vi "WFM MNGR Initialize RF Waveforms.vi"(8 "error in (no error)":errorcluster, 10 "Sequence File":refnum<k7>, 11 "WFM MNGR in":refnum<class "QPA MSMT Waveform Manager.lvclass">) -> (0 "error out":errorcluster, 3 "WFM MNGR out":refnum<class "QPA MSMT Waveform Manager.lvclass">)   [LabVIEW 2016, in "QPA MSMT Waveform Manager.lvclass"]
uses:
  QPA MSMT Waveform Manager.lvclass
  Controls/RF Waveform.ctl
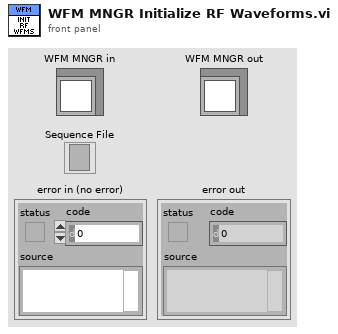
[diagram p1: front panel]
types:
  T1 = typedef "QPA MSMT Waveform Manager.lvclass/RF Waveform.ctl" = cluster{"Name":string, "Path":path, "Headroom":dbl, "Burst Length":dbl}
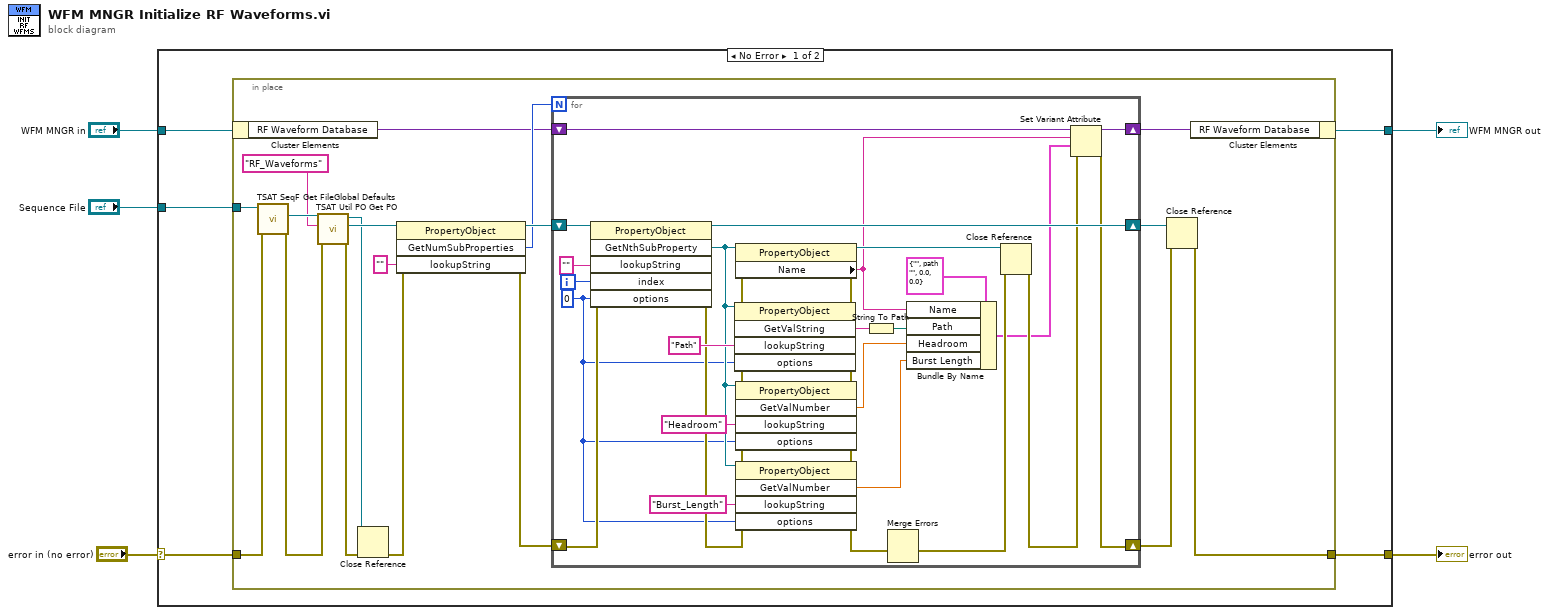
[diagram p0: block diagram]
diagram:
  n1 = case shown="No Error" "error in (no error)" {
    selector: "error in (no error)" -> [w9 w58]
    tunnel: [w6 w58] -> w4
    tunnel: [w7 w57] -> w2
    tunnel: "WFM MNGR in" -> [w8 w57]
    tunnel: "Sequence File" -> [w10 _]
    frame No Error {
      n2 = in-place {
        in-place-border: w10 -> [w17]
        in-place-border: w9 -> [w16]
        in-place-border: [w15] -> w6
        n3 = in-place-cluster #1(w8) -> ("RF Waveform Database"=w14:variant)
        n4 = call "TSAT SeqF Get FileGlobal Defaults.vi"("Error In"=w16, "Sequence File In"=w17) -> ("Error Out"=w26:errorcluster, "FileGlobalsDefaultValues"=w28:refnum<k7>)  [unwired: 7 in, 1 out]
        n5 = call "TSAT Util PO Get PO.vi"("error in (no error)"=w26, "Sub Property to Retrieve"="RF_Waveforms", "Property Object in"=w28) -> ("error out"=w24:errorcluster, "SubProperty"=w25:refnum<k7>, "PropertyObjectOut"=w11:refnum<k7>)  [unwired: 6 in]
        n6 = Close Reference(reference=w11, error in (no error)=w24) -> (error out=w12:errorcluster)
        n7 = invoke class="PropertyObject" method="GetNumSubProperties"(reference=w25, error in=w12, "lookupString"="") -> (reference out=w22:refnum<k7>, error out=w19:errorcluster, "GetNumSubProperties"=w21:i32)  [unwired: 1 in, 1 out]
        n8 = for {
          N: w21 -> [_]
          shift-right: [w54] -> w20
          shift-left: w22 -> [w55]
          shift-right: [w31] -> w18
          shift-left: w19 -> [w53]
          shift-right: [w33] -> w13
          shift-left: w14 -> [w34]
          i -> [w56]
          w40 = 0 ("options")
          n9 = invoke class="PropertyObject" method="GetNthSubProperty"(reference=w55, error in=w53, "lookupString"="", "index"=w56, "options"=w40) -> (reference out=w54:refnum<k7>, error out=w43:errorcluster, "GetNthSubProperty"=w44:refnum<k7>)  [unwired: 1 in, 3 out]
          n10 = invoke class="PropertyObject" method="GetValString"(reference=w44, error in=w43, "lookupString"="Path", "options"=w40) -> (error out=w37:errorcluster, "GetValString"=w48:string)  [unwired: 1 in, 3 out]
          n11 = property class="PropertyObject"(reference=w44, error in=w43) -> (reference out=w51:refnum<k7>, error out=w38:errorcluster, "Name"=w29:string)
          n12 = invoke class="PropertyObject" method="GetValNumber"(reference=w44, error in=w43, "lookupString"="Headroom", "options"=w40) -> (error out=w36:errorcluster, "GetValNumber"=w46:dbl)  [unwired: 1 in, 3 out]
          n13 = invoke class="PropertyObject" method="GetValNumber"(reference=w44, error in=w43, "lookupString"="Burst_Length", "options"=w40) -> (error out=w35:errorcluster, "GetValNumber"=w42:dbl)  [unwired: 1 in, 3 out]
          n14 = String To Path(string=w48) -> (path=w49:path)
          n15 = Merge Errors(w38, w37, w36, w35) -> (w39:errorcluster)
          n16 = Bundle By Name(cluster=T1 {"Name"="", "Path"=path "", "Headroom"=0.0, "Burst Length"=0.0} ("RF Waveform"), "Name"=w29, "Path"=w49, "Headroom"=w46, "Burst Length"=w42) -> (w30:T1)
          n17 = Close Reference(reference=w51, error in (no error)=w39) -> (error out=w32:errorcluster)
          n18 = Set Variant Attribute(Variant=w34, name=w29, value=w30, error in=w32) -> (Variant out=w33:variant, error out=w31:errorcluster)  [unwired: 1 out]
        }
        n19 = Close Reference(reference=w20, error in (no error)=w18) -> (error out=w15:errorcluster)
        n20 = in-place-cluster #1("RF Waveform Database"=w13) -> (w7:refnum<class "QPA MSMT Waveform Manager.lvclass">)
      }
    }
    frame Error {
    }
  }
  "error out" <- w4
  "WFM MNGR out" <- w2
